vi "In Future.vi"(5 "Py":ext, 7 "Px":ext, 11 "Line":T1) -> (3 "Future?":bool)   [LabVIEW 2021]
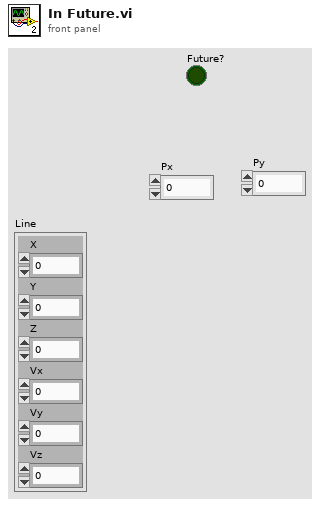
[diagram p1: front panel]
types:
  T1 = cluster{"X":ext, "Y":ext, "Z":ext, "Vx":ext, "Vy":ext, "Vz":ext}
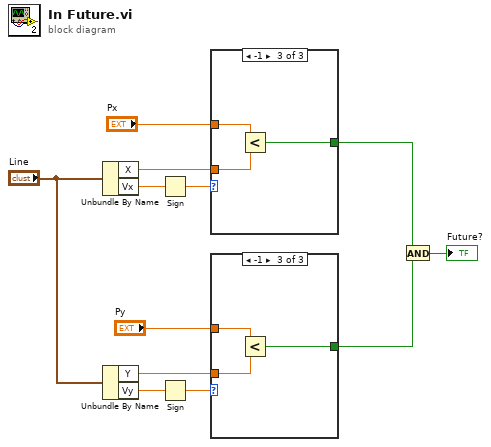
[diagram p0: block diagram]
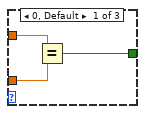
[diagram p2: hidden frame]
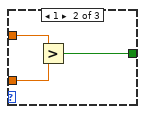
[diagram p3: hidden frame]
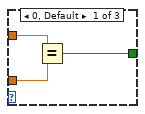
[diagram p4: hidden frame]
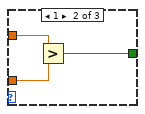
[diagram p5: hidden frame]
diagram:
  n1 = Unbundle By Name("Line") -> ("X"=w9:ext, "Vx"=w12:ext)
  n2 = Unbundle By Name("Line") -> ("Y"=w8:ext, "Vy"=w6:ext)
  n3 = Sign(1:w12) -> (0:w11:ext)
  n4 = Sign(1:w6) -> (0:w7:ext)
  n5 = case shown="-1" w11 {
    tunnel: "Px" -> [w14 w18 w21]
    tunnel: w9 -> [w15 w17 w20]
    tunnel: [w13 w16 w19] -> w2
    frame 0, Default {
      n6 = Equal?(x=w14, y=w15) -> (x = y?=w13:bool)
    }
    frame 1 {
      n7 = Greater?(x=w18, y=w17) -> (0:w16:bool)
    }
    frame -1 {
      n8 = Less?(x=w21, y=w20) -> (x < y?=w19:bool)
    }
  }
  n9 = case shown="-1" w7 {
    tunnel: "Py" -> [w23 w27 w30]
    tunnel: w8 -> [w24 w26 w29]
    tunnel: [w22 w25 w28] -> w3
    frame 0, Default {
      n10 = Equal?(x=w23, y=w24) -> (x = y?=w22:bool)
    }
    frame 1 {
      n11 = Greater?(x=w27, y=w26) -> (0:w25:bool)
    }
    frame -1 {
      n12 = Less?(x=w30, y=w29) -> (x < y?=w28:bool)
    }
  }
  n13 = And(x=w2, y=w3) -> (x .and. y?=→"Future?":bool)
